vi "Read Thermocouples.vi"(0 "task in":refnum<k21>, 5 "tdms file":refnum<k34>, 11 "Error In":errorcluster) -> (4 "task out":refnum<k21>, 6 "Ambient Temp":dbl[unit]=273.15, 8 "Manifold Temp":dbl[unit]=273.15, 10 "Tube Temp":dbl[unit]=273.15, 15 "Error Out":errorcluster)   [LabVIEW 2018]
uses:
  <vilib>/DAQmx/read.llb/DAQmx Read (Analog 1D DBL NChan 1Samp).vi
  <vilib>/DAQmx/miscellaneous.llb/DAQmx Fill In Error Info.vi
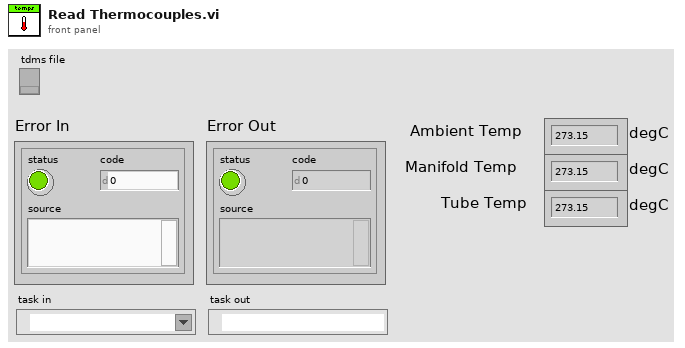
[diagram p1: front panel]
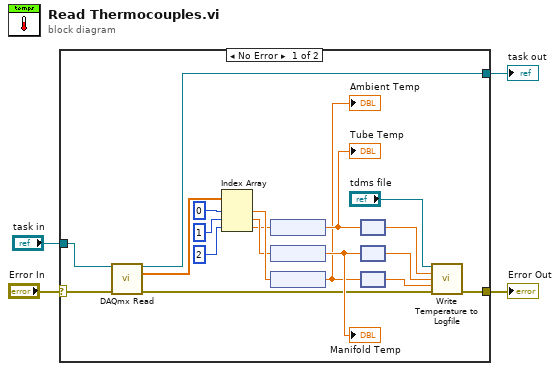
[diagram p0: block diagram]
diagram:
  n1 = case shown="No Error" "Error In" {
    selector: "Error In" -> [w14 w25]
    tunnel: [w10 w25] -> w3
    tunnel: "task in" -> [w15 w24]
    tunnel: [w16 w24] -> w1
    frame No Error {
      n2 = call-poly <vilib>:"DAQmx Read.vi"("task/channels in"=w15, "error in"=w14) -> ("task out"=w16:refnum<k21>, "data"=w23:dbl[], "error out"=w8:errorcluster)  [unwired: 11 in]
      n3 = Index Array(array=w23, index #1=0 ("index"), index #2=1 ("index"), index #3=2 ("index")) -> (element #1=w19:dbl, element #2=w18:dbl, element #3=w17:dbl)
      n4 = node(w17) -> (w13:dbl[unit])
      "Tube Temp" <- w13
      n5 = node(w18) -> (w12:dbl[unit])
      "Manifold Temp" <- w12
      n6 = node(w19) -> (w11:dbl[unit])
      "Ambient Temp" <- w11
      n7 = node(w13) -> (w7:dbl)
      n8 = node(w12) -> (w6:dbl)
      n9 = node(w11) -> (w5:dbl)
      n10 = call "Write Temperature to Logfile.vi"("tdms file"="tdms file", "Tube Temperature (K)"=w7, "Manifold Temperature (K)"=w6, "Ambient Temperature (K)"=w5, "error in (no error)"=w8) -> ("error out"=w10:errorcluster)  [unwired: 9 in, 1 out]
    }
    frame Error {
    }
  }
  "Error Out" <- w3
  "task out" <- w1
